vi "Shuffle Table.vi"(8 "#Cols":i32=3, 9 "#Rows":i32=10, 10 "Tbl Refnum":refnum<vi>, 11 "Array In":string[](array[string])) -> ()   [LabVIEW 2012]
doc: "This VI creates an <B>#Rows</B> by <B>#Cols</B> array and then pushes <B>Array In</B> (which must be 1 by <B>#Cols</B>) into the first position of the array and moves the next <B>#Rows</B> -1 elements into the remaining cells thus creating what is essentially a lossy running table of the data streaming in."
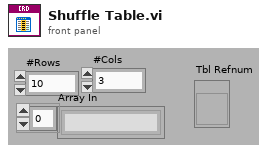
[diagram p1: front panel]
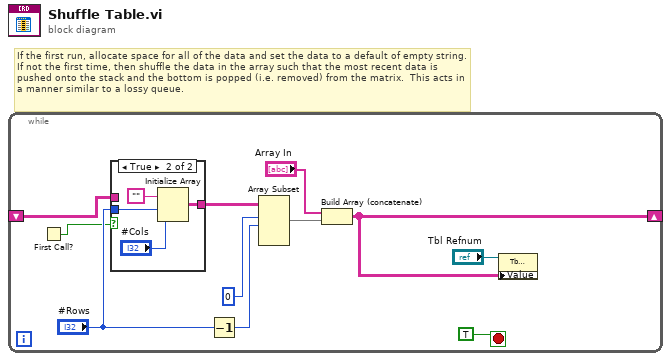
[diagram p0: block diagram]
diagram:
  # "If the first run, allocate space for all of the data and set the data to a default of empty string.  If not the first time, then shuffle the data in the array such that the most recent data is pushed onto the stack and the bottom is popped (i.e. removed) from the matrix.  This acts in a manner similar to a lossy queue."
  n1 = while {
    shift-right: [w5] -> _
    shift-left: _ -> [w4]
    stop <- TRUE ("stop") stop-if-true
    n2 = First Call?() -> (First Call?: T/F=w1:bool)
    n3 = case shown="True" w1 {
      tunnel: [w12 w14] -> w3
      tunnel: "#Rows" -> [_ w13]
      tunnel: w4 -> [w12 _]
      frame False {
      }
      frame True {
        n4 = Initialize Array("", w13, "#Cols") -> (w14:string[][])
      }
    }
    n5 = Decrement(x="#Rows") -> (x-1=w10:i32)
    n6 = Array Subset(array=w3, index (row)=0 ("index"), length (row)=w10) -> (w9:string[][])  [unwired: 2 in]
    n7 = Build Array (concatenate)("Array In", w9) -> (w5:string[][])
    n8 = property class="Tbl (strict)"(reference="Tbl Refnum", "Value"=w5) -> ()  [unwired: 1 in, 2 out]
  }
